vi "logo_in.vi"() -> ()   [LabVIEW 2018]
panel:
  in  "?":bool
  in  "密码:":string="123456"
  in  "帐号:":string="admin"
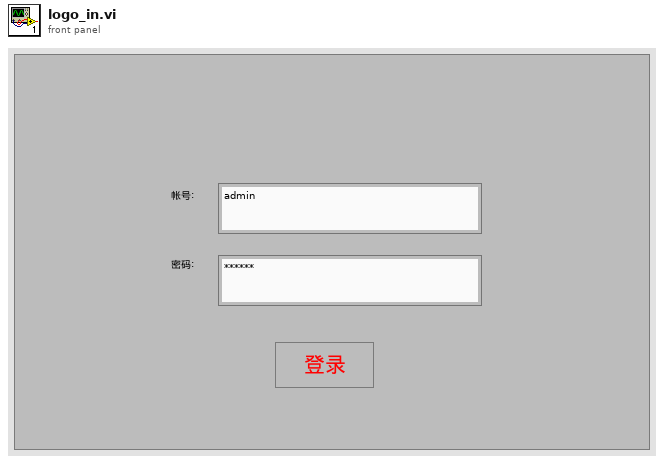
[diagram p1: front panel]
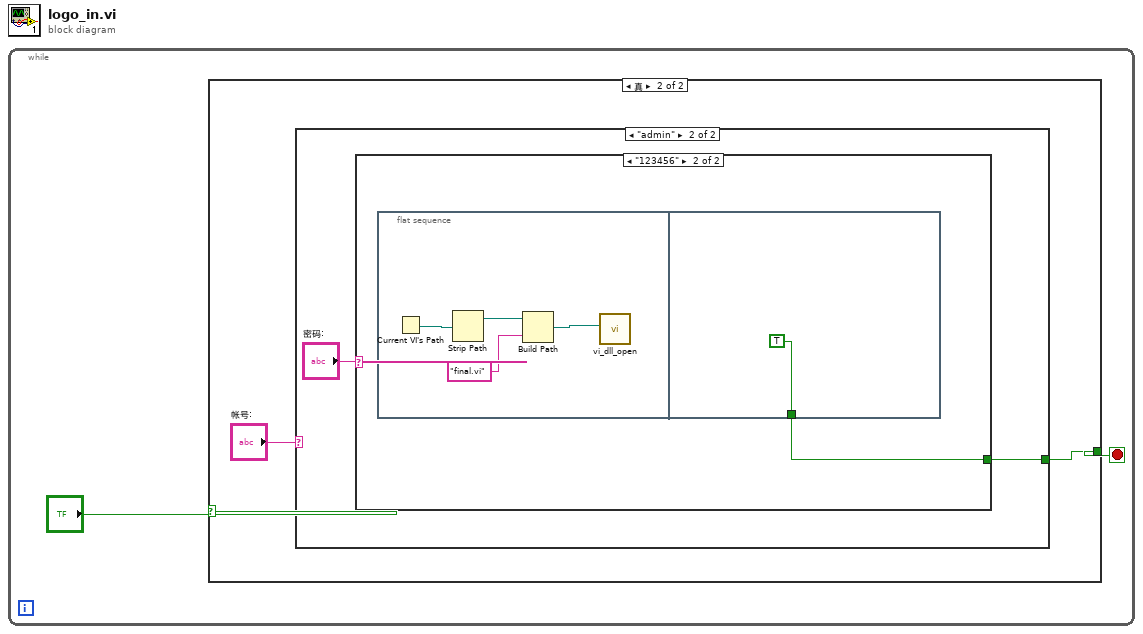
[diagram p0: block diagram]
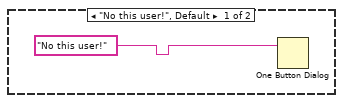
[diagram p3: hidden frame]
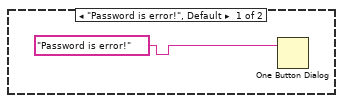
[diagram p4: hidden frame]
diagram:
  n1 = while {
    stop <- w1 stop-if-true
    n2 = case shown="真" "?" {
      tunnel: [_ w3] -> w1
      frame False {
      }
      frame True {
        n3 = case shown="\"admin\"" "帐号:" {
          tunnel: [_ w6] -> w3
          frame "No this user!", Default {
            n4 = One Button Dialog(message="No this user!") -> ()  [unwired: 1 in, 1 out]
          }
          frame "admin" {
            n5 = case shown="\"123456\"" "密码:" {
              tunnel: [_ w9] -> w6
              frame "Password is error!", Default {
                n6 = One Button Dialog(message="Password is error!") -> ()  [unwired: 1 in, 1 out]
              }
              frame "123456" {
                n7 = flat-sequence {
                  tunnel: [TRUE] -> w9
                  frame #0 {
                    n8 = Current VI's Path() -> (path=w12:path)
                    n9 = Strip Path(path=w12) -> (stripped path=w13:path)  [unwired: 1 out]
                    n10 = Build Path(base path=w13, name or relative path="final.vi" ("名称或相对路径")) -> (appended path=w11:path)
                    n11 = call "vi_dll_open.vi"("VI路径"=w11) -> ()  [unwired: 11 in]
                  }
                  frame #1 {
                  }
                }
              }
            }
          }
        }
      }
    }
  }
